vi "Initialize.vi"(8 "error in (no error)":errorcluster, 9 "Power time":dbl=0.15 format="%#_13g", 11 "Container in":refnum<class "Container.lvclass">) -> (0 "error out":errorcluster, 3 "Container out":refnum<class "Container.lvclass">)   [LabVIEW 2016, in "Container.lvclass"]
uses:
  Container.lvclass
  ExtFlat/ExtFlatShutt.lvclass
  SimFlat/SimFlatShutt.lvclass
  LFCSim/LFCSimShutt.lvclass
  Solar/CalShutt.lvclass
  Sci/SciShutt.lvclass
  Container.lvclass/Container.ctl
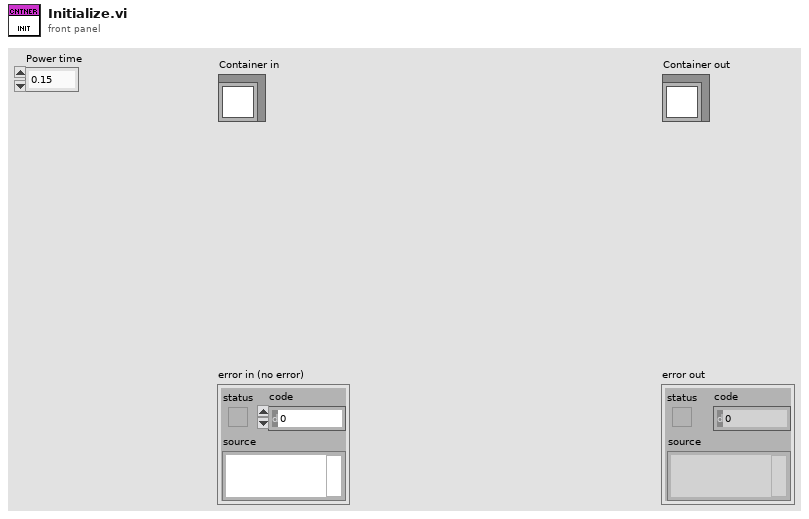
[diagram p1: front panel]
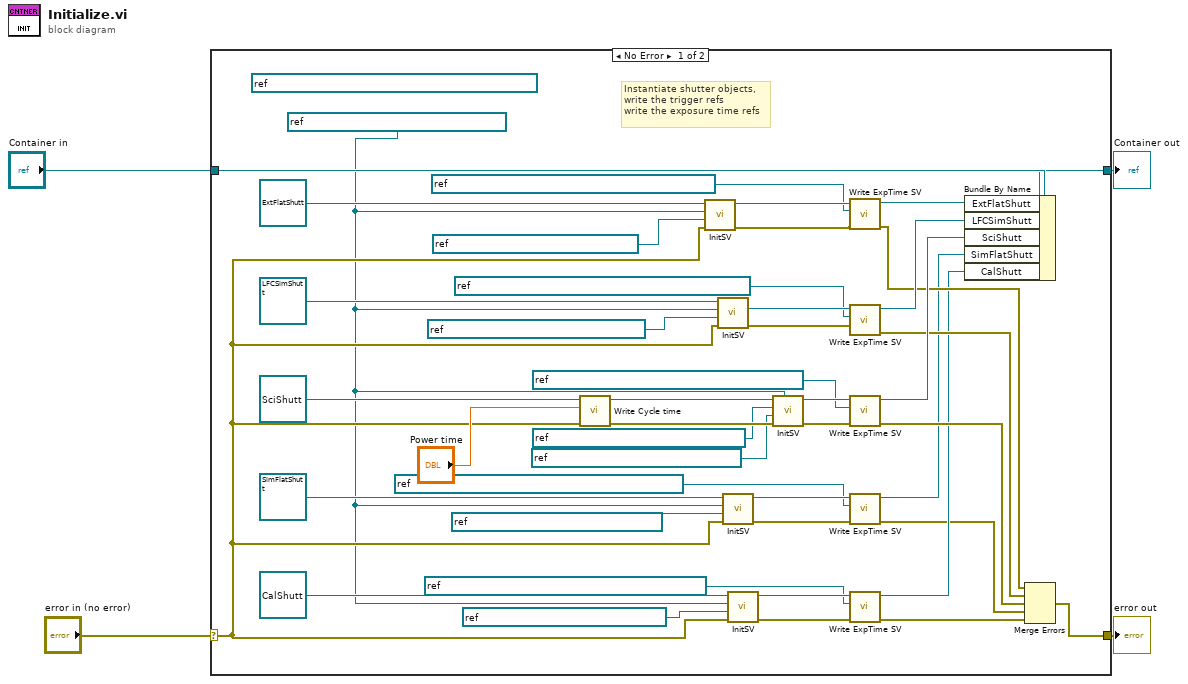
[diagram p0: block diagram]
diagram:
  n1 = case shown="No Error" "error in (no error)" {
    selector: "error in (no error)" -> [w36 w50]
    tunnel: [w37 w50] -> w3
    tunnel: "Container in" -> [w48 w49]
    tunnel: [w47 w49] -> w1
    frame No Error {
      w5 = refnum<k21> "ni.var.psp://bem-rt/Mod2/DetTrigIn" ("TriggerSV refnum")
      (unwired) refnum<k21> "ni.var.psp://bem-rt/RT-Variables/Manaul Trigger" ("TriggerSV refnum")
      # "Instantiate shutter objects,\nwrite the trigger refs\nwrite the exposure time refs"
      n2 = call-dynamic "Write Cycle time.vi"("error in (no error)"=w36, "Power time"="Power time", "BiStableShutter in"=refnum<class "SciShutt.lvclass"> refnum ("SciShutt.lvclass")) -> ("error out"=w39:errorcluster, "BiStableShutter out"=w42:refnum<class "SciShutt.lvclass">)  [unwired: 7 in]
      n3 = call-dynamic "InitSV.vi"("error in (no error)"=w36, "PowerSV refnum"=refnum<k21> "ni.var.io://bem-rt/Mod4/ExtFltSht" ("Power refnum"), "TriggerSV refnum"=w5, "UniStableShutter in"=refnum<class "ExtFlatShutt.lvclass"> refnum ("ExtFlatShutt.lvclass")) -> ("error out"=w20:errorcluster, "UniStableShutter out"=w22:refnum<class "ExtFlatShutt.lvclass">)  [unwired: 6 in]
      n4 = call-dynamic "InitSV.vi"("error in (no error)"=w36, "PowerSV refnum"=refnum<k21> "ni.var.io://bem-rt/Mod4/LFCSimSht", "TriggerSV refnum"=w5, "UniStableShutter in"=refnum<class "LFCSimShutt.lvclass"> refnum ("LFCSimShutt.lvclass")) -> ("error out"=w26:errorcluster, "UniStableShutter out"=w23:refnum<class "LFCSimShutt.lvclass">)  [unwired: 6 in]
      n5 = call-dynamic "InitSV.vi"("error in (no error)"=w36, "PowerSV refnum"=refnum<k21> "ni.var.io://bem-rt/Mod4/SimFltSht", "TriggerSV refnum"=w5, "UniStableShutter in"=refnum<class "SimFlatShutt.lvclass"> refnum ("SimFlatShutt.lvclass")) -> ("error out"=w14:errorcluster, "UniStableShutter out"=w12:refnum<class "SimFlatShutt.lvclass">)  [unwired: 6 in]
      n6 = call-dynamic "InitSV.vi"("error in (no error)"=w36, "PowerSV refnum"=refnum<k21> "ni.var.io://bem-rt/Mod4/SolarSht", "TriggerSV refnum"=w5, "UniStableShutter in"=refnum<class "CalShutt.lvclass"> refnum ("SolarShutt.lvclass")) -> ("error out"=w17:errorcluster, "UniStableShutter out"=w18:refnum<class "CalShutt.lvclass">)  [unwired: 6 in]
      n7 = call-dynamic "InitSV.vi"("TriggerSV refnum"=w5, "error in (no error)"=w39, "Direction refnum"=refnum<k21> "ni.var.io://bem-rt/Mod3/SciShtPol" ("Power refnum"), "Power refnum"=refnum<k21> "ni.var.io://bem-rt/Mod3/SciShtPwr", "BiStableShutter in"=w42) -> ("error out"=w28:errorcluster, "BiStableShutter out"=w30:refnum<class "SciShutt.lvclass">)  [unwired: 5 in]
      n8 = call-dynamic "Write ExpTime SV.vi"("error in (no error)"=w20, "ExpTime SV"=refnum<k21> "ni.var.psp://bem-rt/RT-Variables/ExtFlt Exp Time", "Integrator in"=w22) -> ("error out"=w19:errorcluster, "Integrator out"=w21:refnum<class "ExtFlatShutt.lvclass">)  [unwired: 7 in]
      n9 = call-dynamic "Write ExpTime SV.vi"("error in (no error)"=w26, "ExpTime SV"=refnum<k21> "ni.var.psp://bem-rt/RT-Variables/LFCSim Exp Time", "Integrator in"=w23) -> ("error out"=w25:errorcluster, "Integrator out"=w24:refnum<class "LFCSimShutt.lvclass">)  [unwired: 7 in]
      n10 = call-dynamic "Write ExpTime SV.vi"("error in (no error)"=w28, "ExpTime SV"=refnum<k21> "ni.var.psp://bem-rt/RT-Variables/Sci Exp Time", "Integrator in"=w30) -> ("error out"=w27:errorcluster, "Integrator out"=w29:refnum<class "SciShutt.lvclass">)  [unwired: 7 in]
      n11 = call-dynamic "Write ExpTime SV.vi"("error in (no error)"=w14, "ExpTime SV"=refnum<k21> "ni.var.psp://bem-rt/RT-Variables/SimFlt Exp Time", "Integrator in"=w12) -> ("error out"=w13:errorcluster, "Integrator out"=w11:refnum<class "SimFlatShutt.lvclass">)  [unwired: 7 in]
      n12 = call-dynamic "Write ExpTime SV.vi"("error in (no error)"=w17, "ExpTime SV"=refnum<k21> "ni.var.psp://bem-rt/RT-Variables/Solar Exp Time", "Integrator in"=w18) -> ("error out"=w15:errorcluster, "Integrator out"=w16:refnum<class "CalShutt.lvclass">)  [unwired: 7 in]
      n13 = Bundle By Name(cluster=w48, "ExtFlatShutt"=w21, "LFCSimShutt"=w24, "SciShutt"=w29, "SimFlatShutt"=w11, "CalShutt"=w16) -> (w47:refnum<class "Container.lvclass">)
      n14 = Merge Errors(w19, w25, w27, w13, w15) -> (w37:errorcluster)
    }
    frame Error {
    }
  }
  "error out" <- w3
  "Container out" <- w1
